vi "Elevator Controller Interactive Check.vi"(8 "Interactive Command in":T1={"Operation"=enum."Reserve", "Manual Input"=0.0, "Position"=enum."Bottom Pannel", "1/3 Power"=FALSE}, 9 "Default Command":T1={"Operation"=enum."Reserve", "Manual Input"=0.0, "Position"=enum."Bottom Pannel", "1/3 Power"=FALSE}, 11 "Buttons":cluster{"Execute Cmd":bool, "Abort Cmd":bool}) -> (1 "Interactive Command out":T1={"Operation"=enum."Reserve", "Manual Input"=0.0, "Position"=enum."Bottom Pannel", "1/3 Power"=FALSE}, 2 "Trace String":string, 3 "Schedule":bool)   [LabVIEW 2018]
doc: "Check the Execute and Abort buttons and choose the data and trace string."
uses:
  Elevator Setpoints.ctl
  Elevator Operations.ctl
  Positions.ctl
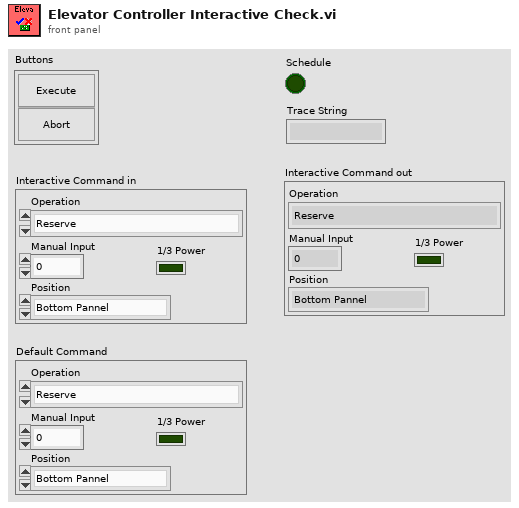
[diagram p1: front panel]
types:
  T1 = typedef "Elevator Setpoints.ctl" = cluster{"Operation":T2, "Manual Input":dbl, "Position":T3, "1/3 Power":bool}
  T2 = typedef "Elevator Operations.ctl" = enum16{"Reserve", "Read Current", "Immediate"}
  T3 = typedef "Positions.ctl" = enum16{"MANUAL", "Bottom Pannel", "Bottom Cargo", "Feeder Station", "Cargo Ship Cargo", "Middle Pannel", "Middle Cargo", "Top Pannel", "Top Cargo"}
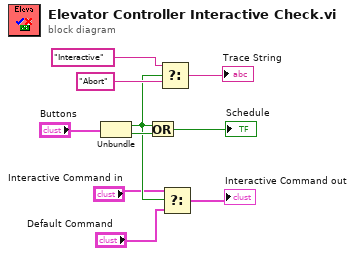
[diagram p0: block diagram]
diagram:
  n1 = Unbundle("Buttons") -> ("Execute Cmd"=w6:bool, "Abort Cmd"=w7:bool)
  n2 = Or(x=w6, y=w7) -> (x .or. y?=→"Schedule":bool)
  n3 = Select(t="Interactive", s=w6, f="Abort") -> (s? t:f=→"Trace String":string)
  n4 = Select(t="Interactive Command in", s=w6, f="Default Command") -> (s? t:f=→"Interactive Command out":T1)
